vi "Peek.vi"(8 "error in (no error)":errorcluster, 11 "Signaller in":refnum<class "Signaller.lvclass">) -> (0 "error out":errorcluster, 2 "Has signal":bool, 3 "Signaller out":refnum<class "Signaller.lvclass">)   [LabVIEW 2015, in "Signaller.lvclass"]
uses:
  Signaller.lvclass
  Signaller.lvclass/Signaller.ctl
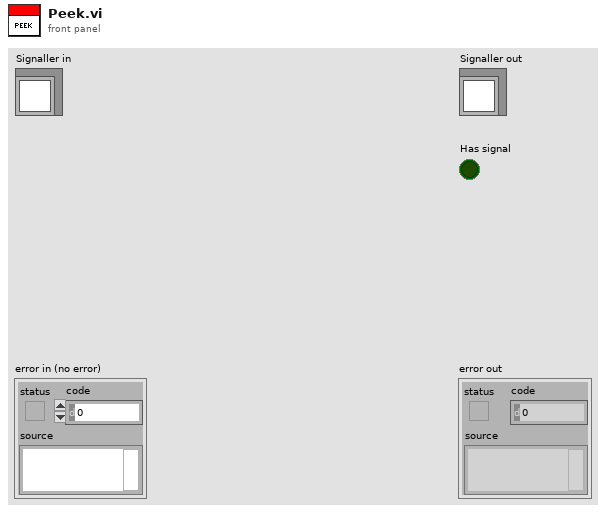
[diagram p1: front panel]
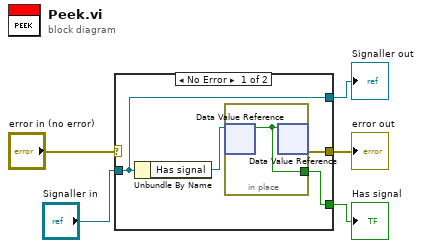
[diagram p0: block diagram]
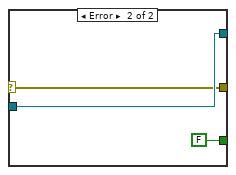
[diagram p2: hidden frame]
diagram:
  n1 = case shown="No Error" "error in (no error)" {
    selector: "error in (no error)" -> [_ w12]
    tunnel: [w6 w12] -> w4
    tunnel: [w9 w13] -> w2
    tunnel: "Signaller in" -> [w9 w13]
    tunnel: [w7 FALSE ("Boolean")] -> w1
    frame No Error {
      n2 = Unbundle By Name(w9) -> ("Has signal"=w8:refnum<data-value>)
      n3 = in-place {
        in-place-border: [w10] -> w7
        n4 = in-place-dvr #1(w8) -> (w10:bool)  [unwired: 1 out]
        n5 = in-place-dvr #1(w10) -> (w6:errorcluster)  [unwired: 1 out]
      }
    }
    frame Error {
    }
  }
  "error out" <- w4
  "Signaller out" <- w2
  "Has signal" <- w1
